vi "SetAttributeViBoolean_Advanced.vi"(7 "AttributeValue (Off)":bool, 8 "error in (no error)":errorcluster {"code" format="%.0x"}, 9 "AttributeID":u32(ring)=1950002 items=["IVILXISYNC_ARM_ALARM_ENABLED"=1950002, "IVILXISYNC_ARM_SOURCE_ENABLED"=1950011, "IVILXISYNC_ARM_SOURCE_OR_ENABLED"=1950014, "IVILXISYNC_EVENT_LOG_ENABLED"=1950034, "IVILXISYNC_TRIGGER_ALARM_ENABLED"=1950016, "LEVEL_ELECTRONIC_ATTENUATION_ENABLED"=1150583, "MARKER_ENABLED"=1250204, "MARKER_FREQUENCY_COUNTER_ENABLED"=1250205, "OUTPUT_ANALOG_AUTO_TYPE_ENABLED"=1150680, "PRESELECTOR_MW_ENABLED"=1150586, "RESOLUTION_BANDWIDTH_AUTO"=1250014, "SIGNAL_TRACK_ENABLED"=1250211, "SIMULATE"=1050005, "STATETRIGGER_ENABLED"=1150160, "SWEEP_MODE_CONTINUOUS"=1250015, "SWEEP_TIME_AUTO"=1250017, "SWEEP_TIME_ENABLED"=1150747, "SYSTEM_TRACE_ENABLED"=1150176, "TRACE_DISPLAY_ENABLED"=1150758, "TRACE_UPDATE_ENABLED"=1150757, "TRACES_AVERAGE_ENABLED"=1150756, "TRACES_AVERAGE_TYPE_AUTO_ENABLED"=1150667, "TRIGGER_AUTO__ENABLED"=1150845, "TRIGGER_EXTERNAL2_DELAY_ENABLED "=1150834, "TRIGGER_EXTERNAL_DELAY_ENABLED"=1150835, "TRIGGER_EXTERNAL2_ZERO_SPAN_DELAY_COMPENSATION_ENABLED"=1150808, "TRIGGER_EXTERNAL_ZERO_SPAN_DELAY_COMPENSATION_ENABLED"=1150807, "TRIGGER_FRAME_DELAY_ENABLED"=1150843, "TRIGGER_HOLD_OFF_ENABLED"=1150848, "TRIGGER_LINE_DELAY_ENABLED"=1150838, "TRIGGER_RFBURST_DELAY_ENABLED"=1150832, "TRIGGER_VIDEO_DELAY_ENABLED "=1150833, "VIDEO_BANDWIDTH_AUTO"=1250023, "ZERO_SPAN_DELAY_COMPENSATION_ENABLED"=1150849], 10 "RepCapIdentifier":string, 11 "instrument handle":refnum<k15>) -> (0 "error out":errorcluster {"code" format="%.0x"}, 3 "instrument handle out":refnum<k15>)   [LabVIEW 2009, in "Keysight XSAn.lvlib"]
doc: "Sets a Boolean attribute from the instrument driver.\nThe following Attributes are supported:\n\nIVILXISYNC_ARM_ALARM_ENABLED\nIVILXISYNC_ARM_SOURCE_ENABLED\nIVILXISYNC_ARM_SOURCE_OR_ENABLED\nIVILXISYNC_EVENT_LOG_ENABLED\nIVILXISYNC_TRIGGER_ALARM_ENABLED\nLEVEL_ELECTRONIC_ATTENUATION_ENABLED\nMARKER_ENABLED\nMARKER_FREQUENCY_COUNTER_ENABLED\nOUTPUT_ANALOG_AUTO_TYPE_ENABLED\nPRESELECTOR_MW_ENABLED\nRESOLUTION_BANDWIDTH_AUTO\nSIGNAL_TRACK_ENABLED\nSIMULATE\nSTATETRIGGER_ENABLED\nSWEEP_MODE_CONTINUOUS\nSWEEP_TIME_AUTO\nSWEEP_TIME_ENABLED\nSYSTEM_TRACE_ENABLED\nTRACE_DISPLAY_ENABLED\nTRACE_UPDATE_ENABLED\nTRACES_AVERAGE_ENABLED\nTRACES_AVERAGE_TYPE_AUTO_ENABLED\nTRIGGER_AUTO__ENABLED\nTRIGGER_EXTERNAL2_DELAY_ENABLED\nTRIGGER_EXTERNAL_DELAY_ENABLED\nTRIGGER_EXTERNAL2_ZERO_SPAN_DELAY_COMPENSATION_ENABLED \nTRIGGER_EXTERNAL_ZERO_SPAN_DELAY_COMPENSATION_ENABLED \nTRIGGER_FRAME_DELAY_ENABLED\nTRIGGER_HOLD_OFF_ENABLED\nTRIGGER_LINE_DELAY_ENABLED\nTRIGGER_RFBURST_DELAY_ENABLED\nTRIGGER_VIDEO_DELAY_ENABLED\nVIDEO_BANDWIDTH_AUTO\nZERO_SPAN_DELAY_COMPENSATION_ENABLED"
uses:
  <instrlib>/Keysight XSAn/Keysight XSAn.lvlib
  AgXSAn.dll
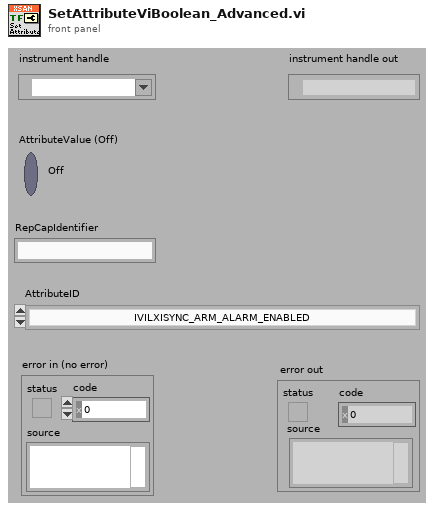
[diagram p1: front panel]
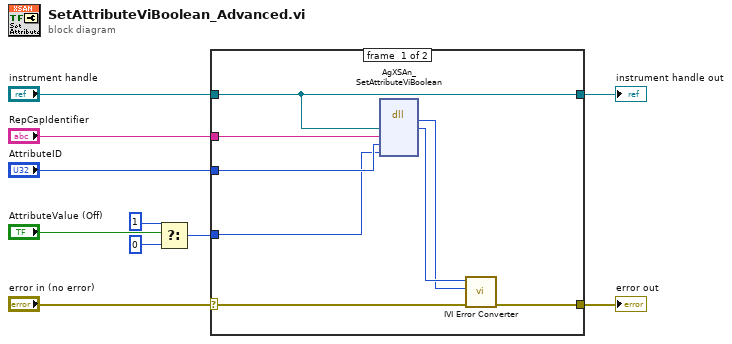
[diagram p0: block diagram]
diagram:
  n1 = Select(t=u16 1, s="AttributeValue (Off)", f=u16 0) -> (s? t:f=w2:u16)
  n2 = case shown="No Error" "error in (no error)" {
    selector: "error in (no error)" -> [w16 w20]
    tunnel: [w15 w20] -> w10
    tunnel: "instrument handle" -> [w11 w19]
    tunnel: "RepCapIdentifier" -> [w14 _]
    tunnel: "AttributeID" -> [w13 _]
    tunnel: w2 -> [w12 _]
    tunnel: [w11 w19] -> w1
    frame #0 {
      n3 = dll-call lib="AgXSAn**.dll" fn="AgXSAn_SetAttributeViBoolean"("Vi"=w11, "RepCapIdentifier"=w14, "AttributeID"=w13, "AttributeValue"=w12) -> ("return type"=w17:i32, "Vi"=w18:u32)  [unwired: 6 in, 2 out]
      n4 = call <instrlib>:"IVI Error Converter.vi"("error in (no error)"=w16, "IVI error code (0)"=w17, "instrument handle"=w18) -> ("error out"=w15:errorcluster)  [unwired: 7 in, 1 out]
    }
    frame #1 {
    }
  }
  "error out" <- w10
  "instrument handle out" <- w1
